vi "Create All Message Queues.vi"(8 "error in (no error)":errorcluster caption="错误输入（无错误）") -> (0 "error out":errorcluster caption="错误输出", 3 "Message Queues out":T1 caption="消息队列输出")   [LabVIEW 2014, in "Message Queue.lvlib"]
doc: "本VI用于创建应用程序所需的所有消息队列。如应用程序需要两个以上消息队列，可右键单击上面的“消息队列”常量并选择“打开自定义类型”，将新的消息队列添加至该自定义类型，然后通过本VI进行初始化。"
uses:
  Message Queue.lvlib
  All Message Queues.ctl
  Message Cluster.ctl
  Enqueue Message (Single).vi
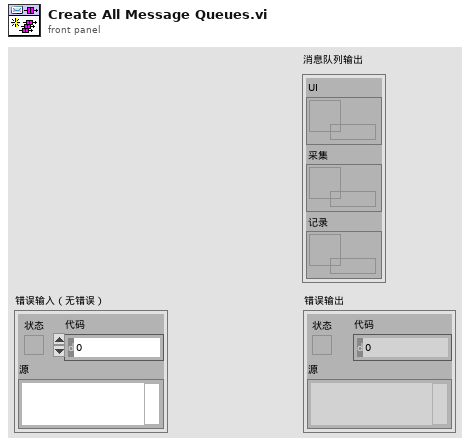
[diagram p1: front panel]
types:
  T1 = typedef "Message Queue.lvlib/All Message Queues.ctl" = cluster{"UI":refnum<queue>, "Acquisition":refnum<queue>, "Logging":refnum<queue>}
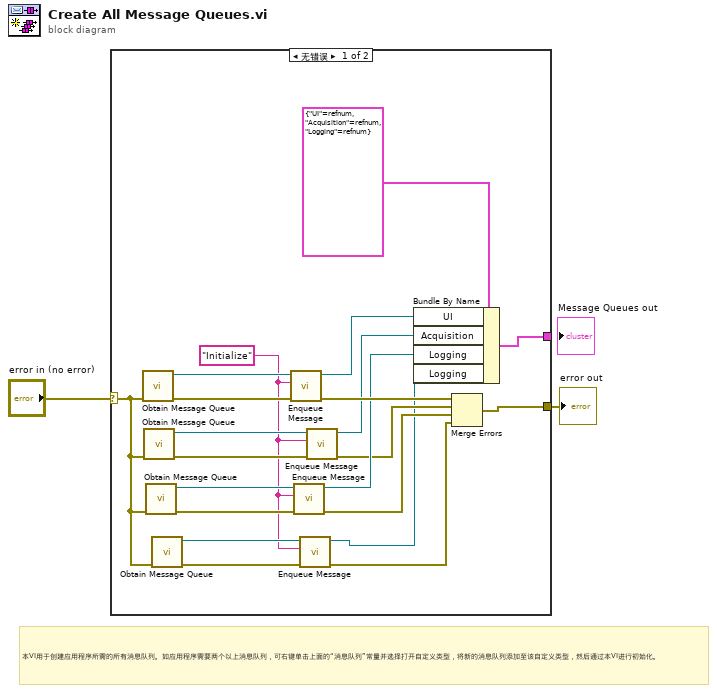
[diagram p0: block diagram]
diagram:
  # "本VI用于创建应用程序所需的所有消息队列。如应用程序需要两个以上消息队列，可右键单击上面的“消息队列”常量并选择打开自定义类型，将新的消息队列添加至该自定义类型，然后通过本VI进行初始化。"
  n1 = case shown="无错误" "error in (no error)" {
    selector: "error in (no error)" -> [w6 w24]
    tunnel: [w12 w24] -> w2
    tunnel: [w22 _] -> _
    frame No Error {
      w5 = "Initialize" ("Message")
      n2 = call "Obtain Message Queue.vi"("error in (no error)"=w6) -> ("error out"=w21:errorcluster, "Message Queue"=w20:refnum<queue>)  [unwired: 9 in]
      n3 = call "Obtain Message Queue.vi"("error in (no error)"=w6) -> ("error out"=w18:errorcluster, "Message Queue"=w19:refnum<queue>)  [unwired: 9 in]
      n4 = call "Obtain Message Queue.vi"("error in (no error)"=w6) -> ("error out"=w17:errorcluster, "Message Queue"=w16:refnum<queue>)  [unwired: 9 in]
      n5 = call "Obtain Message Queue.vi"("error in (no error)"=w6) -> ("error out"=w8:errorcluster, "Message Queue"=w7:refnum<queue>)  [unwired: 9 in]
      n6 = call-poly "Enqueue Message.vi"("error in (no error)"=w21, "Message"=w5, "Message Queue"=w20) -> ("error out"=w23:errorcluster, "dup Message Queue"=w15:refnum<queue>)  [unwired: 7 in]
      n7 = call-poly "Enqueue Message.vi"("error in (no error)"=w17, "Message"=w5, "Message Queue"=w16) -> ("error out"=w10:errorcluster, "dup Message Queue"=w13:refnum<queue>)  [unwired: 7 in]
      n8 = call-poly "Enqueue Message.vi"("error in (no error)"=w8, "Message"=w5, "Message Queue"=w7) -> ("error out"=w4:errorcluster, "dup Message Queue"=w3:refnum<queue>)  [unwired: 7 in]
      n9 = call-poly "Enqueue Message.vi"("error in (no error)"=w18, "Message"=w5, "Message Queue"=w19) -> ("error out"=w11:errorcluster, "dup Message Queue"=w14:refnum<queue>)  [unwired: 7 in]
      n10 = Bundle By Name(cluster=T1 {"UI"=refnum, "Acquisition"=refnum, "Logging"=refnum} ("Message Queues"), "UI"=w15, "Acquisition"=w14, "Logging"=w13, "Logging"=w3) -> (w22:T1)
      n11 = Merge Errors(w23, w11, w10, w4) -> (w12:errorcluster)
    }
    frame Error {
    }
  }
  "error out" <- w2
